vi "Set Param.vi"(2 "error in (no error)":errorcluster, 3 "param":dbl, 4 "paramID":i32) -> (0 "error out":errorcluster, 1 "function return":i32)   [LabVIEW 2014, in "ThorPMT.lvlib"]
doc: "long SetParam(const long paramID, const double param);"
uses:
  ThorPMT.lvlib
  ThorPMT.dll
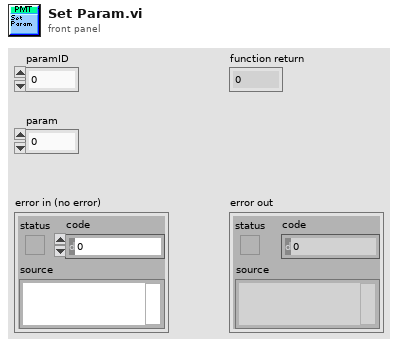
[diagram p1: front panel]
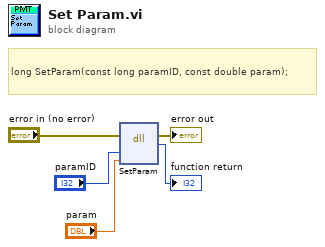
[diagram p0: block diagram]
diagram:
  # "long SetParam(const long paramID, const double param);"
  n1 = dll-call lib="C:/TIS_CalebVS2012/TIS_Development/Hardware/SDKs/PMT_SDK/LabVIEW/inc/ThorPMT.dll" fn="SetParam"(error in="error in (no error)", "paramID"="paramID", "param"="param") -> (error out=→"error out":errorcluster, "return type"=→"function return":i32)  [unwired: 4 in, 1 out]
